vi "S2C_ReadScript.vi"(8 "Error In":errorcluster, 11 "FilePath":path) -> (0 "Error Out":errorcluster, 3 "Data":string[][](array[string]))   [LabVIEW 2015]
doc: "Deletes the selected items from the script table."
uses:
  <vilib>/Utility/config.llb/Read Key (String).vi
  <vilib>/Utility/config.llb/NI_LVConfig.lvlib
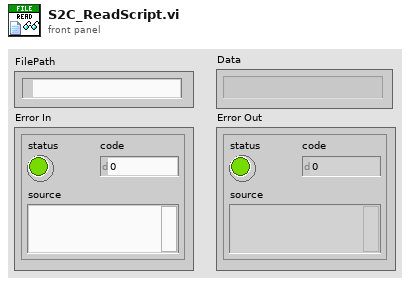
[diagram p1: front panel]
types:
  T1 = typedef "NI_LVConfig.lvlib/Config Data RefNum.ctl" = refnum<k1>
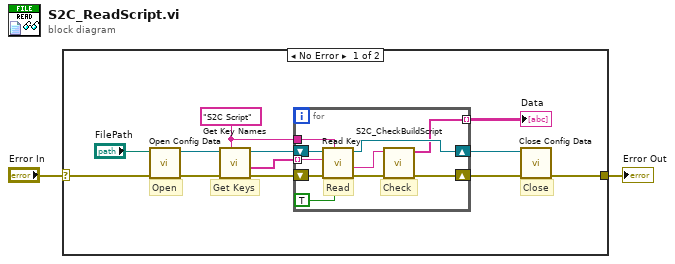
[diagram p0: block diagram]
diagram:
  n1 = case shown="No Error" "Error In" {
    selector: "Error In" -> [w4 w25]
    tunnel: [w6 w25] -> w1
    frame No Error {
      w9 = "S2C Script"
      # "Close"
      # "Get Keys"
      # "Open"
      n2 = call <vilib>:"Open Config Data.vi"("error in (no error)"=w4, "configuration file path"="FilePath") -> ("error out"=w12:errorcluster, "refnum"=w11:T1)  [unwired: 7 in, 1 out]
      n3 = call <vilib>:"Get Key Names.vi"("section"=w9, "error in (no error)"=w12, "refnum"=w11) -> ("error out"=w10:errorcluster, "key names"=w7:string[], "refnum out"=w8:T1)  [unwired: 5 in, 1 out]
      n4 = for {
        shift-right: [w19] -> w14
        shift-left: w10 -> [w24]
        tunnel: w9 -> [w23]
        shift-right: [w18] -> w13
        shift-left: w8 -> [w22]
        tunnel: w7 -> [w21] mode=indexing
        tunnel: [w16] -> w3 mode=indexing
        # "Check"
        # "Read"
        n5 = call-poly <vilib>:"Read Key.vi"("read raw string? (F)"=TRUE, "section"=w23, "error in (no error)"=w24, "key"=w21, "refnum"=w22) -> ("error out"=w20:errorcluster, "value"=w17:string, "refnum out"=w18:T1)  [unwired: 3 in, 1 out]
        n6 = call "S2C_CheckBuildScript.vi"("Error In"=w20, "Entry"=w17) -> ("Error Out"=w19:errorcluster, "Data"=w16:string[])  [unwired: 8 in]
      }
      "Data" <- w3
      n7 = call <vilib>:"Close Config Data.vi"("error in (no error)"=w14, "refnum"=w13) -> ("error out"=w6:errorcluster)  [unwired: 8 in, 1 out]
    }
    frame Error {
    }
  }
  "Error Out" <- w1
